vi "ParseVCLorTXTdir.vi"(8 "error in (no error)":errorcluster, 11 "path in":path) -> (0 "error out":errorcluster, 2 "type":string, 3 "appended path":path[](array[path]))   [LabVIEW 2016, in "VCL_2_DSC.lvclass"]
uses:
  VCL_2_DSC.lvclass
  <userlib>/_OpenG.lib/file/file.llb/Build Path - File Names Array__ogtk.vi
  <userlib>/_OpenG.lib/array/array.llb/Remove Duplicates from 1D Array (String)__ogtk.vi
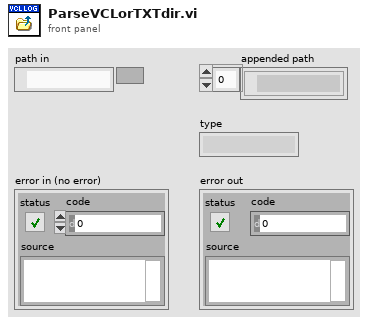
[diagram p1: front panel]
types:
  T1 = enum16{"Left Button", "Center Button", "Right Button", "Window Close"}
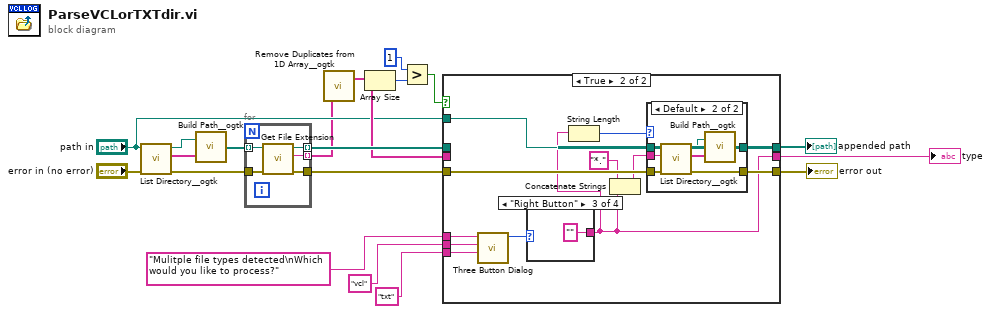
[diagram p0: block diagram]
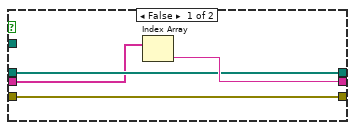
[diagram p2: hidden frame]
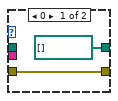
[diagram p3: hidden frame]
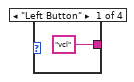
[diagram p4: hidden frame]
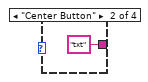
[diagram p5: hidden frame]
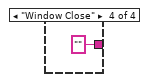
[diagram p6: hidden frame]
diagram:
  n1 = call <userlib>:"List Directory__ogtk.vi"("error in (no error)"="error in (no error)", "directory path"="path in") -> ("error out"=w12:errorcluster, "file names"=w14:string[], "dup directory path"=w11:path)  [unwired: 2 in, 1 out]
  n2 = call-poly <userlib>:"Build Path__ogtk.vi"("name or relative path"=w14, "base path"=w11) -> ("appended path"=w10:path[])
  n3 = for {
    tunnel: w10 -> [w24] mode=indexing
    tunnel: [w23] -> w1 mode=indexing
    tunnel: w12 -> [w22]
    tunnel: [w21] -> w9 mode=indexing
    tunnel: [w20] -> w5
    n4 = call <vilib>:"Get File Extension.vi"("error in (no error)"=w22, "file"=w24) -> ("error out"=w20:errorcluster, "lowercase file extension"=w23:string, "dup file"=w21:path)  [unwired: 5 in, 2 out]
  }
  n5 = call-poly <userlib>:"Remove Duplicates from 1D Array__ogtk.vi"("Input Array"=w1) -> ("Output Array"=w8:string[])  [unwired: 1 out]
  n6 = Array Size(array=w8) -> (size(s)=w15:i32)
  n7 = Greater?(x=1 ("y"), y=w15) -> (0:w17:bool)
  n8 = case shown="True" w17 {
    tunnel: w8 -> [w25 _]
    tunnel: [w28 w31] -> w4
    tunnel: "Mulitple file types detected\nWhich would you like to process?" ("message") -> [_ w40]
    tunnel: "txt" ("message") -> [_ w39]
    tunnel: "vcl" ("message") -> [_ w38]
    tunnel: [w27 w36] -> w19
    tunnel: w9 -> [w27 _]
    tunnel: w5 -> [w26 w35]
    tunnel: [w26 w34] -> w3
    tunnel: "path in" -> [_ w33]
    frame False {
      n9 = Index Array(array=w25) -> (element=w28:string)  [unwired: 1 in]
    }
    frame True {
      n10 = call <vilib>:"Three Button Dialog.vi"("Center Button Text (\"No\")"=w39, "Left Button Text (\"Yes\")"=w38, "message"=w40) -> ("Which Button?"=w37:T1)  [unwired: 8 in]
      n11 = case shown="\"Right Button\"" w37 {
        tunnel: ["vcl" ("String") "txt" ("String") "" ("String") "" ("String")] -> w31
        frame "Left Button" {
        }
        frame "Center Button" {
        }
        frame "Right Button" {
        }
        frame "Window Close" {
        }
      }
      n12 = String Length(string=w31) -> (length=w32:i32)
      n13 = Concatenate Strings("*." ("String"), w31) -> (w30:string)
      n14 = case shown="Default" w32 {
        tunnel: [path[] [] ("appended path") w47] -> w36
        tunnel: w35 -> [w42 w46]
        tunnel: [w42 w45] -> w34
        tunnel: w30 -> [_ w44]
        tunnel: w33 -> [_ w43]
        frame 0 {
        }
        frame Default {
          n15 = call <userlib>:"List Directory__ogtk.vi"("error in (no error)"=w46, "pattern"=w44, "directory path"=w43) -> ("error out"=w45:errorcluster, "file names"=w49:string[], "dup directory path"=w48:path)  [unwired: 1 in, 1 out]
          n16 = call-poly <userlib>:"Build Path__ogtk.vi"("name or relative path"=w49, "base path"=w48) -> ("appended path"=w47:path[])
        }
      }
    }
  }
  "appended path" <- w19
  "type" <- w4
  "error out" <- w3
